vi "test_stat_f_1.vi"() -> ()   [LabVIEW 2010]
panel:
  out "channel name(s) out":string[](array[string])
  out "error out":errorcluster
  in  "file path (dialog if empty)":path
  out "Waveform Graph 3":waveform(i16)[](graph)
  out "t0":timestamp format="%<%.6X>T"
  out "Array 2":timestamp[](array[timestamp]) format="%<%.7X>T"
  out "pieces":i32=1
  in  "piece":i32=1
  out "Waveform Graph 2":waveform(i16)(graph)
  out "Waveform Graph":waveform(dbl)[](graph)
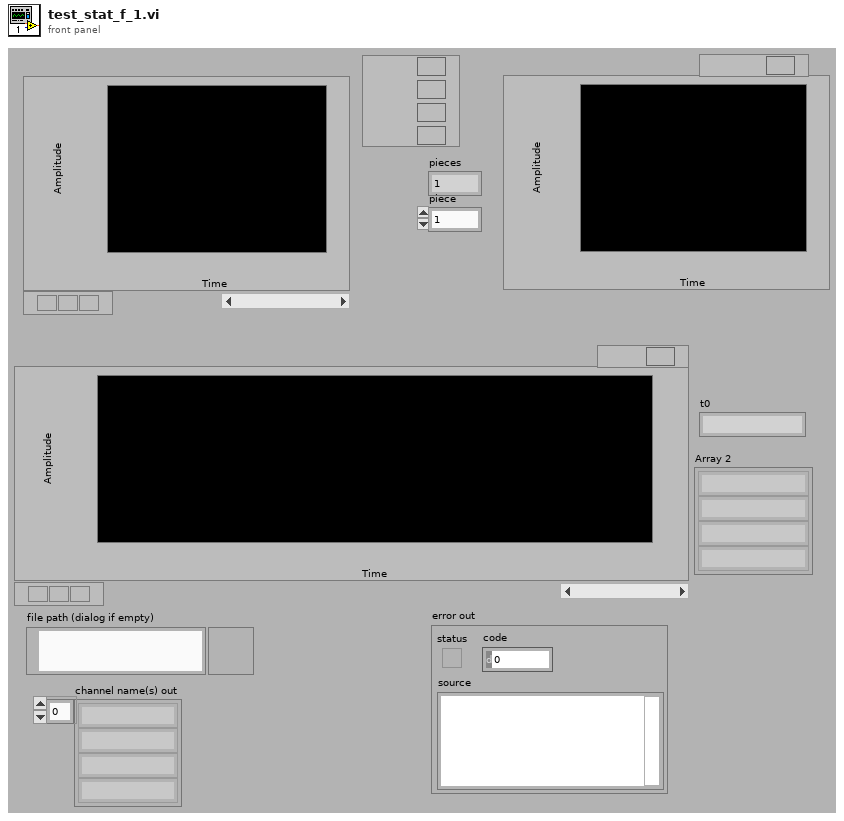
[diagram p1: front panel]
types:
  T1 = cluster{"second":i32, "minute":i32, "hour":i32, "day of month":i32, "month":i32, "year":i32, "day of week":i32, "day of year":i32, "is DST":i32}
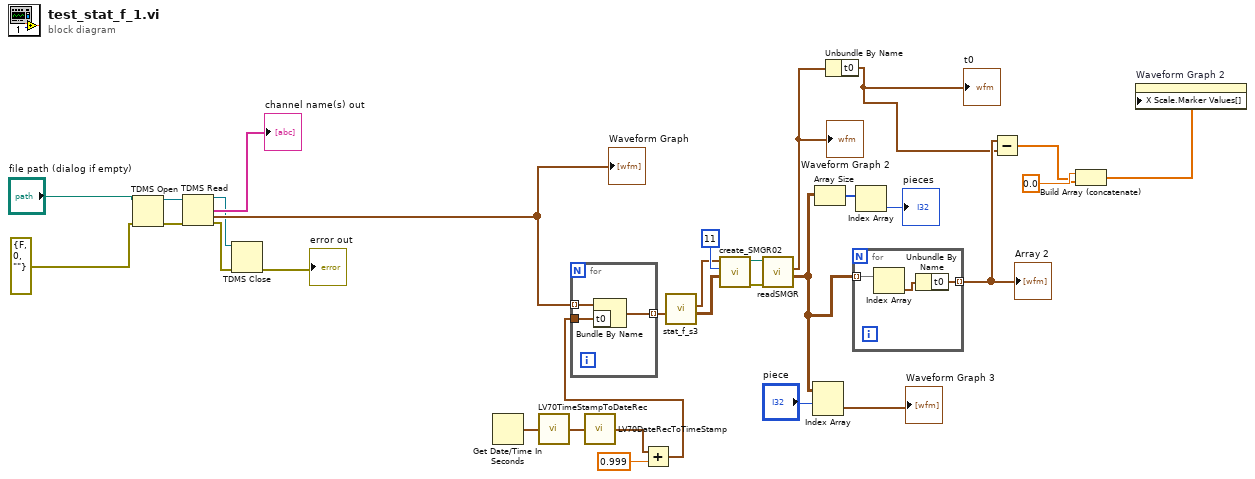
[diagram p0: block diagram]
diagram:
  n1 = TDMS Open(8:errorcluster {"status"=FALSE, "code"=0, "source"=""} ("error in (no error)"), 11:"file path (dialog if empty)") -> (0:w7:errorcluster, 3:w8:refnum<k34>)  [unwired: 4 in]
  n2 = TDMS Read(0:w8, 11:w7) -> (4:w4:refnum<k34>, 8:→"channel name(s) out":string[], 10:w5:waveform(dbl)[], 15:w3:errorcluster)  [unwired: 5 in, 2 out]
  "Waveform Graph" <- w5
  n3 = TDMS Close(8:w3, 11:w4) -> (0:→"error out":errorcluster)  [unwired: 1 out]
  n4 = Get Date/Time In Seconds() -> (seconds since 1Jan1904=w17:timestamp)
  n5 = call <vilib>:"LV70TimeStampToDateRec.vi"("time stamp"=w17) -> ("date time rec"=w15:T1)
  n6 = call <vilib>:"LV70DateRecToTimeStamp.vi"("date time rec"=w15) -> ("Time Stamp"=w14:timestamp)
  n7 = Add(x=w14, y=0.999) -> (x+y=w13:timestamp)
  n8 = for {
    tunnel: w5 -> [w34] mode=indexing
    tunnel: [w33] -> w26 mode=indexing
    tunnel: w13 -> [w32]
    n9 = Bundle By Name(cluster=w34, "t0"=w32) -> (w33:waveform(dbl))
  }
  n10 = call "stat_f_s3.vi"("Array of Waveform"=w26) -> ("Array 2"=w12:waveform(i16)[][], "sync"=w20:waveform(i16))  [unwired: 5 in]
  n11 = call "create_SMGR02.vi"("array"=w12, "meas_point"=11 ("n"), "sync"=w20) -> ("error out"=w30:errorcluster, "path"=w1:path)  [unwired: 3 in]
  n12 = call "readSMGR.vi"("error in"=w30, "file path"=w1) -> ("output array"=w11:waveform(i16)[][], "sync"=w19:waveform(i16))  [unwired: 3 in, 1 out]
  "Waveform Graph 2" <- w19
  n13 = Index Array(array=w11, index (row)="piece") -> (element=→"Waveform Graph 3":waveform(i16)[])  [unwired: 1 in]
  n14 = Array Size(array=w11) -> (size(s)=w28:i32[])
  n15 = Unbundle By Name(w19) -> ("t0"=w24:timestamp)
  "t0" <- w24
  n16 = for {
    tunnel: w11 -> [w37] mode=indexing
    tunnel: [w35] -> w25 mode=indexing
    n17 = Index Array(array=w37) -> (element=w36:waveform(i16))  [unwired: 1 in]
    n18 = Unbundle By Name(w36) -> ("t0"=w35:timestamp)
  }
  "Array 2" <- w25
  n19 = Index Array(array=w28) -> (element=→"pieces":i32)  [unwired: 1 in]
  n20 = Subtract(x=w25, y=w24) -> (x-y=w22:dbl[])
  n21 = Build Array (concatenate)(0.0, w22) -> (w21:dbl[])
  n22 = property on="Waveform Graph 2" class="WFGraph (strict)"("X Scale.Marker Values[]"=w21) -> ()  [unwired: 2 in, 2 out]
